vi "Read Files of SubFolder (Row).vi"(8 "error in (no error)":errorcluster, 10 "RowIndex":i32, 11 "Folder_Mgmt in":refnum<class "Folder_Mgmt.lvclass">) -> (0 "error out":errorcluster, 2 "FolderFiles (Row)":string[](array[string]), 3 "Folder_Mgmt out":refnum<class "Folder_Mgmt.lvclass">)   [LabVIEW 2016, in "Folder_Mgmt.lvclass"]
uses:
  Folder_Mgmt.lvclass
  Folder_Mgmt.lvclass/Folder_Mgmt.ctl
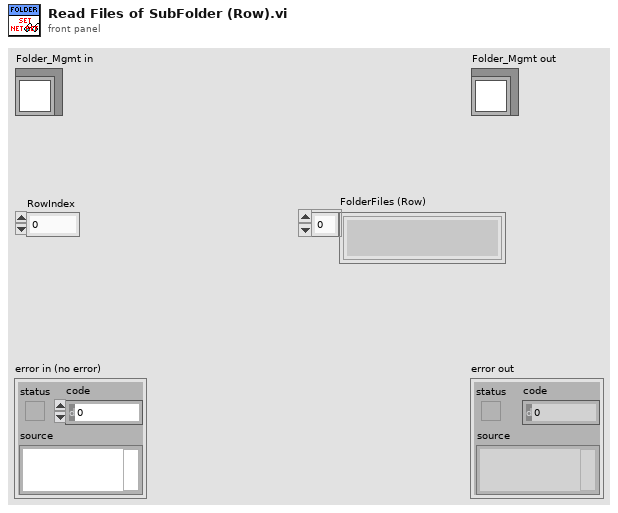
[diagram p1: front panel]
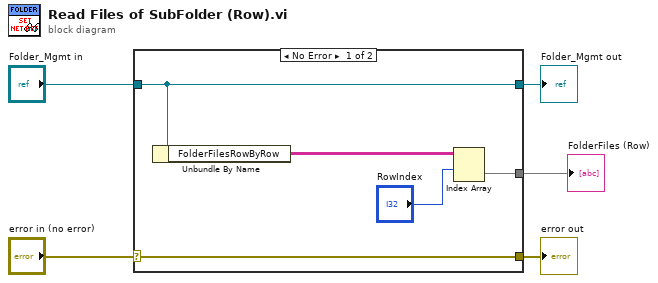
[diagram p0: block diagram]
diagram:
  n1 = case shown="No Error" "error in (no error)" {
    selector: "error in (no error)" -> [w10 w11]
    tunnel: [w10 w11] -> w4
    tunnel: [w9 w12] -> w2
    tunnel: "Folder_Mgmt in" -> [w9 w12]
    tunnel: [w6 _] -> w1
    frame No Error {
      n2 = Unbundle By Name(w9) -> ("FolderFilesRowByRow"=w8:string[][])
      n3 = Index Array(array=w8, index (row)="RowIndex") -> (element=w6:string[])  [unwired: 1 in]
    }
    frame Error {
    }
  }
  "error out" <- w4
  "Folder_Mgmt out" <- w2
  "FolderFiles (Row)" <- w1
